vi "MQTT_Simple_Connect_and_Subscribe.vi"() -> ()   [LabVIEW 2017, in "MQTT_Functions.lvlib"]
doc: "A basic client example that connects to a server, subscribes to a variety of topics and receives responses for the topics. \n\n© 2015 - daq.io, LLC - Peter Adelhardt"
uses:
  MQTT_Functions.lvlib
  Controls/Connect_Flags.ctl
  Controls/QoS.ctl
  Controls/Connection_Return_Codes.ctl
  Controls/MessageType.ctl
  Controls/DUP_Flag.ctl
  Controls/Retain_Flag.ctl
panel:
  out "Messages":T2(array[cluster])
  in  "Stop Reading":bool
  in  "MQTT Broker":cluster{"address (IP)":string, "port":u16}={"address (IP)"="broker.hivemq.com", "port"=1883}
  in  "Subscription Info Array":cluster{"Topic":string, "QoS":T3}[](array[cluster])=[{"Topic"="testtopic/LVMQTT", "QoS"=enum."At most once"}]
  out "Granted QoS Levels":T3[](array[typedef])
  out "Connection Status":T4=enum."Connection refused: Server unavailable"
  in  "Connect Flags":T5
  in  "Client ID":string="LVSubscribeClient"
  out "error out":errorcluster
  in  "error in (no error)":errorcluster
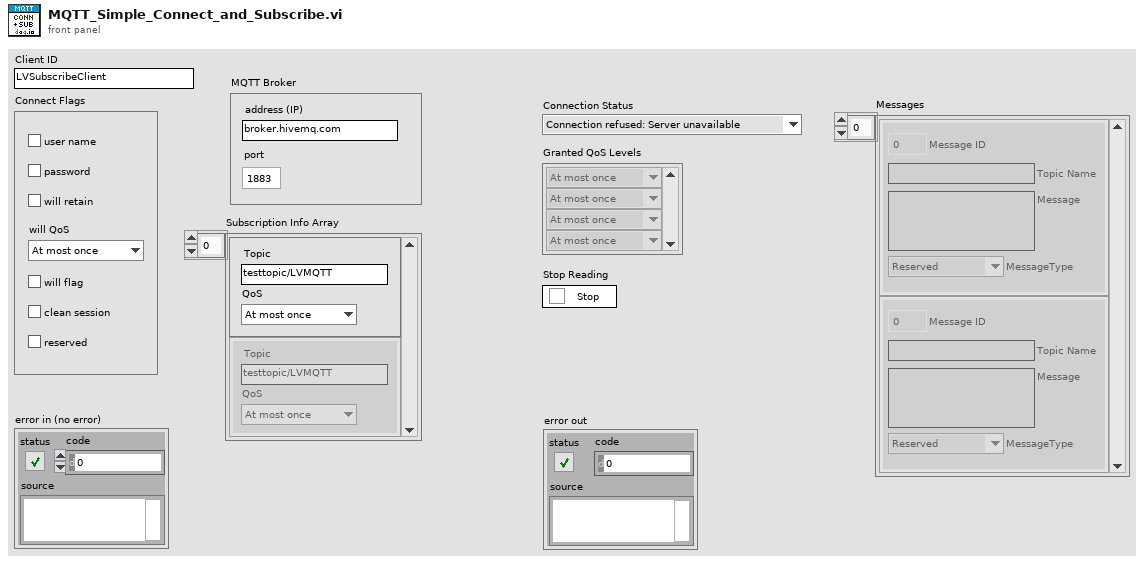
[diagram p1: front panel]
types:
  T1 = typedef "MQTT_Functions.lvlib/MessageType.ctl" = enum32{"Reserved", "CONNECT", "CONNACK", "PUBLISH", "PUBACK", "PUBREC", "PUBREL", "PUBCOMP", "SUBSCRIBE", "SUBACK", "UNSUBSCRIBE", "UNSUBACK", "PINGREQ", "PINGRESP", "DISCONNECT", "Reserved2"}
  T2 = cluster{"Message ID":u16, "Topic Name":string, "Message ":string, "MessageType":T1}[]
  T3 = typedef "MQTT_Functions.lvlib/QoS.ctl" = enum8{"At most once", "At least once", "Exactly once", "Reserved"}
  T4 = typedef "MQTT_Functions.lvlib/Connection_Return_Codes.ctl" = enum16{"Connection accepted", "Connection refused: unacceptable protocol version", "Connection refused: identifier rejected", "Connection refused: Server unavailable", "Connection refused: bad user name or password", "Connection refused: not authorized"}
  T5 = typedef "MQTT_Functions.lvlib/Connect_Flags.ctl" = cluster{"user name":bool, "password":bool, "will retain":bool, "will flag":bool, "clean session":bool, "reserved":bool, "will QoS":T3}
  T6 = cluster{"Message ID":u16, "Topic Name":string, "Message":string, "MessageType":T1}[]
  T7 = typedef "MQTT_Functions.lvlib/DUP_Flag.ctl" = bool
  T8 = typedef "MQTT_Functions.lvlib/Retain_Flag.ctl" = bool
  T9 = cluster{"QoS":T3, "DUP":T7, "Retain":T8, "Keep Alive (sec)":u16}
  T10 = cluster{"Message ID":u16, "Topic Name":string, "Message":string, "MessageType":T1}
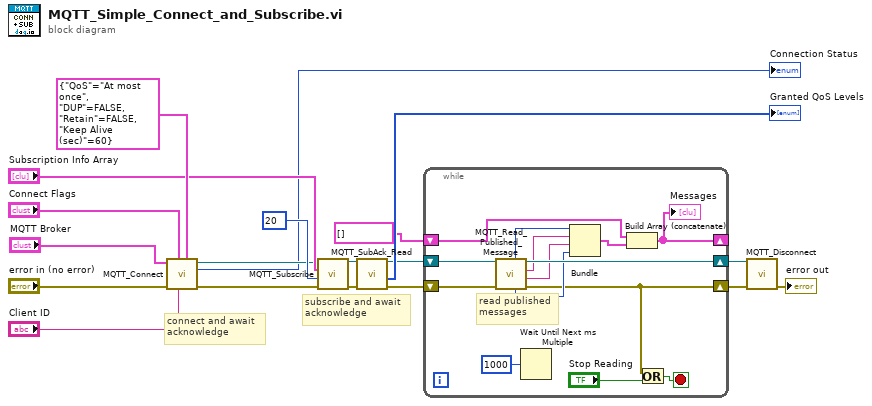
[diagram p0: block diagram]
diagram:
  # "connect and await\nacknowledge"
  # "subscribe and await\nacknowledge"
  n1 = call "MQTT_Connect.vi"("Connect Meta"=T9 {"QoS"=enum."At most once", "DUP"=FALSE, "Retain"=FALSE, "Keep Alive (sec)"=60}, "Client ID"="Client ID", "Connect Flags"="Connect Flags", "error in (no error)"="error in (no error)", "MQTT Broker"="MQTT Broker") -> ("error out"=w1:errorcluster, "Connection Status"=→"Connection Status":T4, "connection ID out"=w3:refnum<k5>)  [unwired: 4 in]
  n2 = call "MQTT_Subscribe.vi"("error in (no error)"=w1, "Message ID"=u16 20, "Subscription Info Array"="Subscription Info Array", "connection ID"=w3) -> ("error out"=w12:errorcluster, "connection ID out"=w13:refnum<k5>)  [unwired: 6 in]
  n3 = call "MQTT_SubAck_Read.vi"("error in (no error)"=w12, "connection ID"=w13) -> ("error out"=w10:errorcluster, "Granted QoS Levels"=→"Granted QoS Levels":T3[], "connection ID out"=w9:refnum<k5>)  [unwired: 7 in]
  n4 = while {
    shift-right: [w20] -> _
    shift-left: T6 [] ("Array") -> [w22]
    shift-right: [w23] -> w7
    shift-left: w10 -> [w33]
    shift-right: [w31] -> w8
    shift-left: w9 -> [w32]
    stop <- w25 stop-if-true
    # "read published\nmessages"
    n5 = call "MQTT_Read_Published_Message.vi"("error in (no error)"=w33, "connection ID"=w32) -> ("error out"=w23:errorcluster, "Message"=w28:string, "Topic Name"=w29:string, "connection ID out"=w31:refnum<k5>, "MessageType"=w27:T1, "Message ID"=w30:u16)  [unwired: 4 in]
    n6 = Wait Until Next ms Multiple(millisecond multiple=u32 1000) -> ()  [unwired: 1 out]
    n7 = Bundle("Message ID"=w30, "Topic Name"=w29, "Message"=w28, "MessageType"=w27) -> (w21:T10)  [unwired: 1 in]
    n8 = Build Array (concatenate)(w22, w21) -> (w20:T6)
    "Messages" <- w20
    n9 = Or(x=w23, y="Stop Reading") -> (x .or. y?=w25:bool)
  }
  n10 = call "MQTT_Disconnect.vi"("error in (no error)"=w7, "connection ID"=w8) -> ("error out"=→"error out":errorcluster)  [unwired: 9 in]
